vi "Increment Limits Popup.vi"(8 "error in (no error)":errorcluster) -> (0 "error out":errorcluster)   [LabVIEW 2009]
uses:
  lib/Data Access Objects/Metadata/LBCB Number.ctl
  lib/Data Access Objects/Metadata/Cartesian Point.ctl
  Update Actions.ctl
  lib/Data Access Objects/Metadata/DAO Actions.ctl
  lib/Data Access Objects/Metadata/Persistant DAO Actions.ctl
panel:
  out "Current Increments":dbl[](array[numeric])=[-0.014471871278962644, -0.0027477897622864888, 0.03594582291831433, -0.006177356244415369, -0.000527948512754489, 0.04718526152757189]
  in  "Ok":bool
  in  "Increment Limits":T1
  in  "LBCB Number":T2
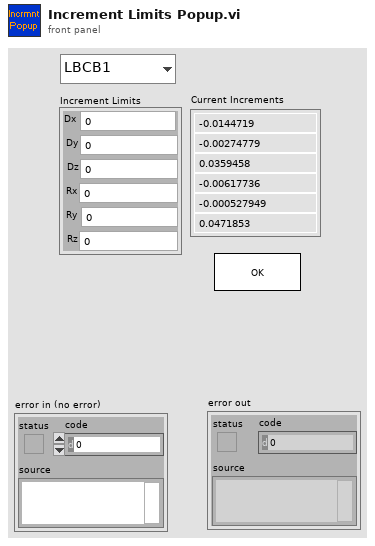
[diagram p1: front panel]
types:
  T1 = typedef "Cartesian Point.ctl" = cluster{"Dx":dbl, "Dy":dbl, "Dz":dbl, "Rx":dbl, "Ry":dbl, "Rz":dbl}
  T2 = typedef "LBCB Number.ctl" = enum16{"LBCB1", "LBCB2"}
  T3 = typedef "Update Actions.ctl" = enum16{"Update", "Exit"}
  T4 = typedef "DAO Actions.ctl" = enum16{"Init", "Get", "Set"}
  T5 = typedef "Persistant DAO Actions.ctl" = enum16{"Init", "Get", "Set", "Load", "Save"}
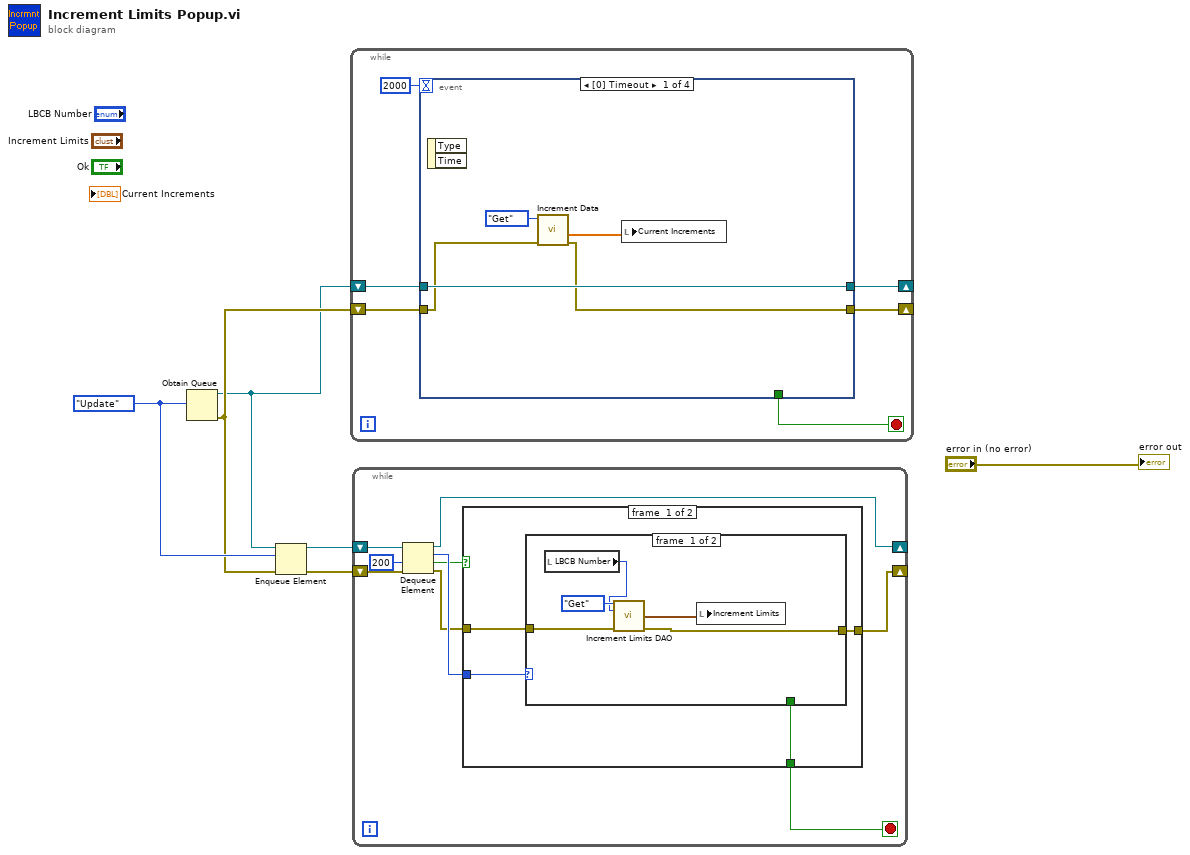
[diagram p0: block diagram]
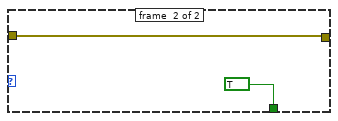
[diagram p2: hidden frame]
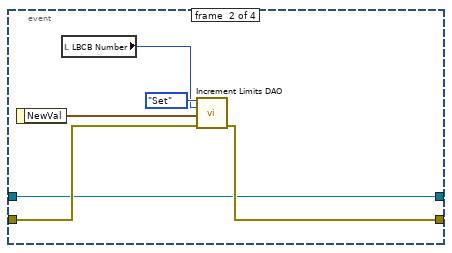
[diagram p4: hidden frame]
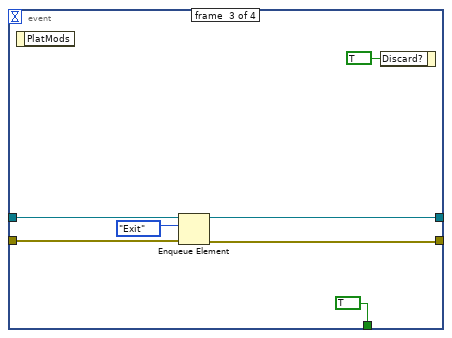
[diagram p5: hidden frame]
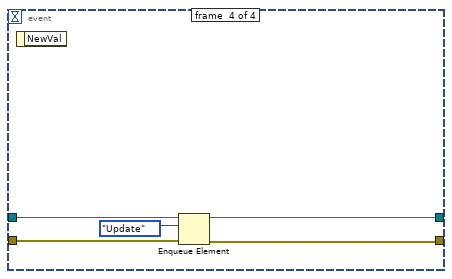
[diagram p6: hidden frame]
diagram:
  w4 = Update_Actions."Update" ("Update Actions")
  n1 = Obtain Queue(element data type=w4) -> (queue out=w2:refnum<queue>, error out=w3:errorcluster)  [unwired: 4 in, 1 out]
  n2 = Enqueue Element(queue=w2, element=w4, error in (no error)=w3) -> (queue out=w6:refnum<queue>, error out=w5:errorcluster)  [unwired: 1 in, 1 out]
  n3 = while {
    shift-right: [w10] -> _
    shift-left: w3 -> [w11]
    shift-right: [w8] -> _
    shift-left: w2 -> [w9]
    stop <- w7 stop-if-true
    n4 = event shown="[0] Timeout" {
      selector: _ -> [_ _ _ _]
      dyn-events: _ -> [_ _ _ _]
      timeout: 2000 -> [_ _ _ _]
      tunnel: w11 -> [w14 w20 w30 w35]
      tunnel: [w13 w19 w29 w34] -> w10
      tunnel: w9 -> [w17 w18 w28 w33]
      tunnel: [w17 w18 w26 w32] -> w8
      tunnel: [_ _ TRUE _] -> w7
      event #0 {
        n5 = event-data() -> ()  [unwired: 1 in, 2 out]
        n6 = call "Increment Data.vi"("error in (no error)"=w14, "DAO Actions"=DAO_Actions."Get") -> ("error out"=w13:errorcluster, "Increments Out"=w15:dbl[])  [unwired: 8 in]
        n7 = local write "Current Increments"(w15) -> ()
      }
      event #1 {
        n8 = event-data() -> ("NewVal"=w23:T1)  [unwired: 1 in]
        n9 = local read "LBCB Number"() -> (w21:T2)
        n10 = call "Increment Limits DAO.vi"("Actions"=Persistant_DAO_Actions."Set", "LBCB Number"=w21, "Inc Limits In"=w23, "error in (no error)"=w20) -> ("error out"=w19:errorcluster)  [unwired: 9 in, 2 out]
      }
      event #2 {
        n11 = event-data() -> ()  [unwired: 1 in, 1 out]
        n12 = Enqueue Element(queue=w28, element=Update_Actions."Exit", error in (no error)=w30) -> (queue out=w26:refnum<queue>, error out=w29:errorcluster)  [unwired: 1 in, 1 out]
        n13 = event-data("Discard?"=TRUE) -> ()  [unwired: 1 in, 1 out]
      }
      event #3 {
        n14 = event-data() -> ()  [unwired: 1 in, 1 out]
        n15 = Enqueue Element(queue=w33, element=Update_Actions."Update", error in (no error)=w35) -> (queue out=w32:refnum<queue>, error out=w34:errorcluster)  [unwired: 1 in, 1 out]
      }
    }
  }
  n16 = while {
    shift-right: [w41] -> _
    shift-left: w6 -> [w44]
    shift-right: [w38] -> _
    shift-left: w5 -> [w43]
    stop <- w37 stop-if-true
    n17 = Dequeue Element(queue=w44, timeout in ms (-1)=200, error in (no error)=w43) -> (queue out=w41:refnum<queue>, element=w40:T3, timed out?=w36:bool, error out=w39:errorcluster)
    n18 = case shown="False" w36 {
      tunnel: w40 -> [w48 _]
      tunnel: w39 -> [w47 w56]
      tunnel: [w46 w56] -> w38
      tunnel: [w45 _] -> w37
      frame #0 {
        n19 = case shown="\"Update\"" w48 {
          tunnel: w47 -> [w50 w55]
          tunnel: [w49 w55] -> w46
          tunnel: [_ TRUE] -> w45
          frame #0 {
            n20 = local read "LBCB Number"() -> (w52:T2)
            n21 = call "Increment Limits DAO.vi"("Actions"=Persistant_DAO_Actions."Get", "LBCB Number"=w52, "error in (no error)"=w50) -> ("Inc Limits Out"=w51:T1, "error out"=w49:errorcluster)  [unwired: 10 in, 1 out]
            n22 = local write "Increment Limits"(w51) -> ()
          }
          frame #1 {
          }
        }
      }
      frame #1 {
      }
    }
  }
  "error out" <- "error in (no error)"
